vi "CRYUnflatten Scope-FFT.vi"(11 "Flat Scope-FFT setup":string) -> (0 "Error?":bool=TRUE, 2 "Scope-FFT settings":T1={"window"=0, "n avgs"=0, "lin/exp avg"=0, "pwr/cplx avg"=0, "time (ms)"=0.0, "fft lines"=2048, "scope/fft mode"=0, "channel"=0, "trig. channel"=0, "Applay Correction"=FALSE, "Time Display"="%#_6p", "Freq. Weighting"="%.1f", "Ave/Max/Min"=0, "Trigger Level"=0.0, "Trigger Unit"=0, "Trigger Time Offset"=0.0, "Trigger Slope"=0, "Trigger/Free Run"=FALSE, "continuous"=FALSE, "Spectrum Display"="%#_6p", "Calc FFT"=FALSE, "Y-axis"="None", "Signal Type"=""} {"Trigger Time Offset" format="%.2f"; "Trigger Level" format="%.2f"; "time (ms)" format="%.2f"}, 3 "Header info":T2={"Data type"="Data            ", "Version"=1, "Dimensions"=0})   [LabVIEW 2013]
uses:
  Typedef Control/CRYScope-FFT.ctl
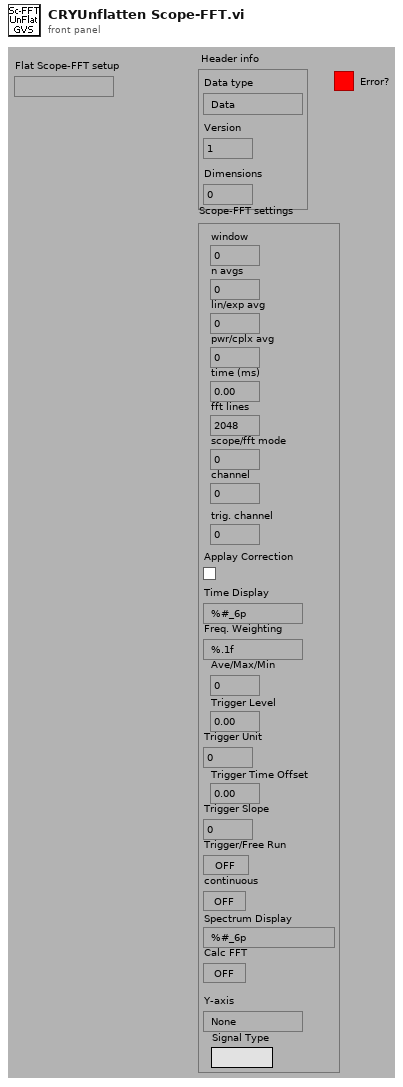
[diagram p1: front panel]
types:
  T1 = typedef "CRYScope-FFT.ctl" = cluster{"window":i32, "n avgs":i32, "lin/exp avg":i32, "pwr/cplx avg":i32, "time (ms)":dbl, "fft lines":i32, "scope/fft mode":i32, "channel":i32, "trig. channel":i32, "Applay Correction":bool, "Time Display":string, "Freq. Weighting":string, "Ave/Max/Min":u16, "Trigger Level":dbl, "Trigger Unit":u16, "Trigger Time Offset":dbl, "Trigger Slope":u16, "Trigger/Free Run":bool, "continuous":bool, "Spectrum Display":string, "Calc FFT":bool, "Y-axis":string, "Signal Type":string}
  T2 = cluster{"Data type":string, "Version":u16, "Dimensions":u8}
  T3 = cluster{"unsigned byte array[0]":u8, "unsigned byte array[1]":u8, "unsigned byte array[2]":u8}
  T4 = cluster{"substring":string, u16, "unsigned byte array[2]":u8}
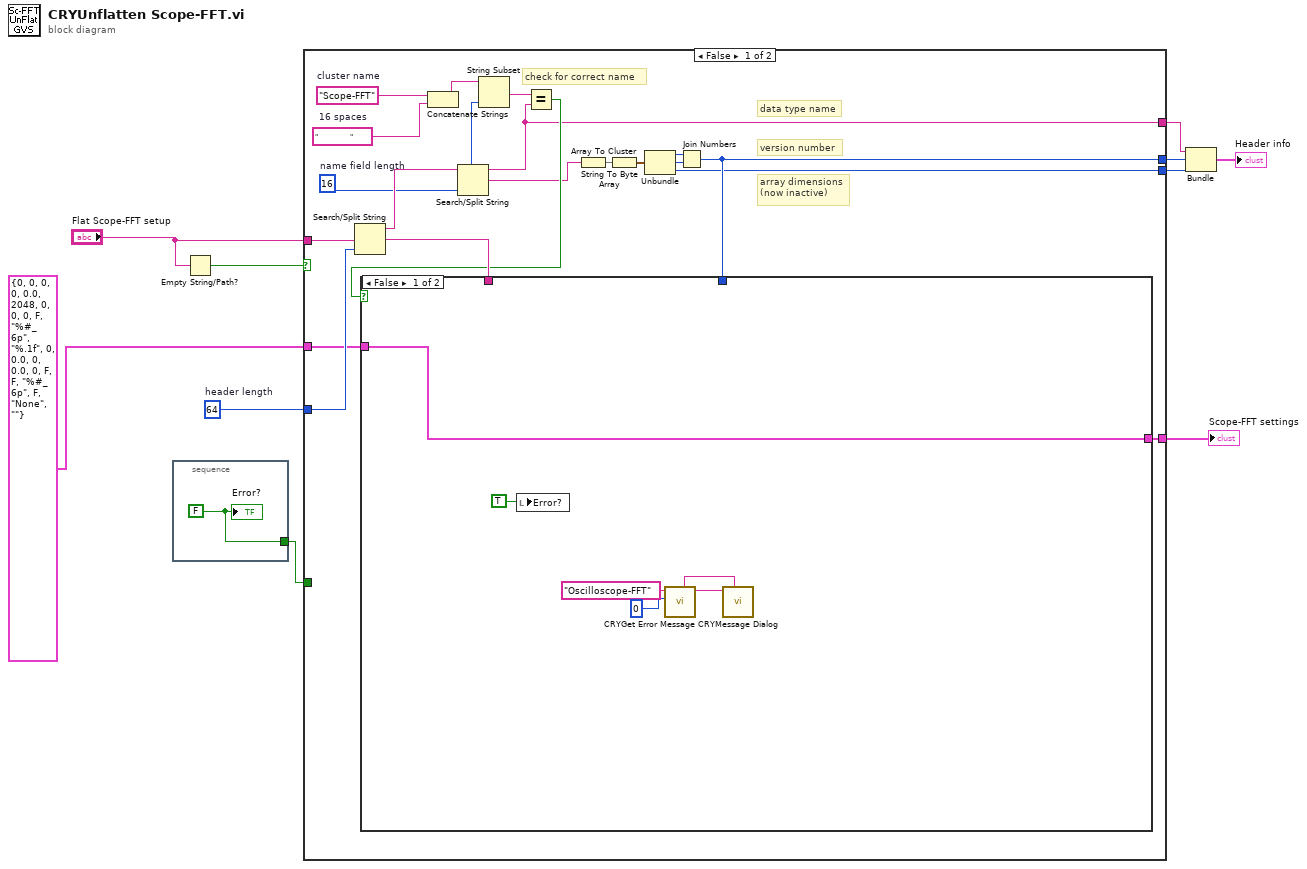
[diagram p0: block diagram]
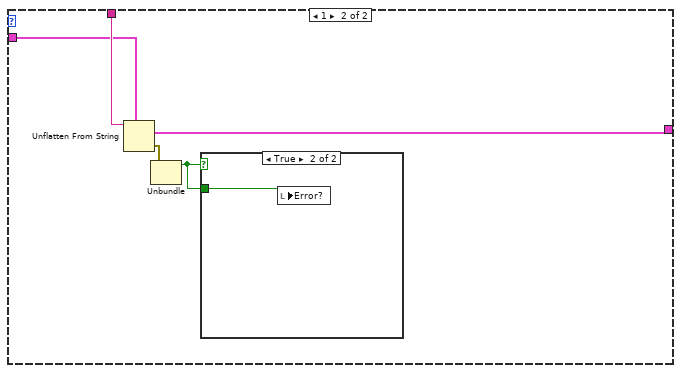
[diagram p3: hidden frame]
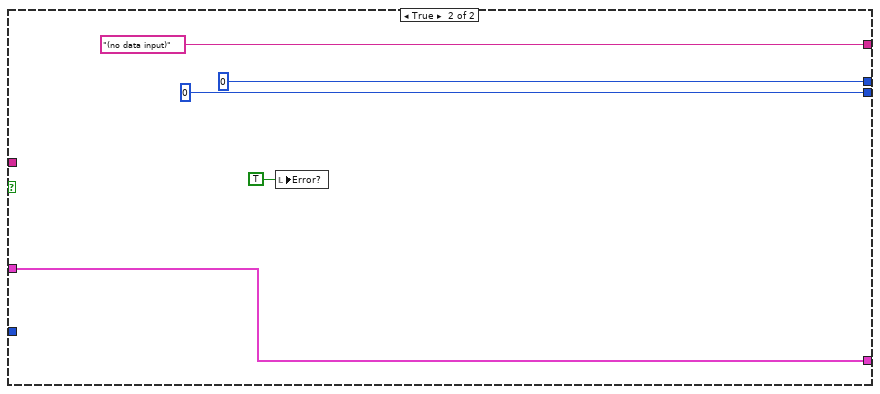
[diagram p5: hidden frame]
diagram:
  w9 = 64  # header length
  n1 = stacked-sequence {
    tunnel: [w11] -> w5
    frame #0 {
      w11 = FALSE
      "Error?" <- w11
    }
  }
  n2 = Empty String/Path?(string/path="Flat Scope-FFT setup") -> (empty?=w10:bool)
  n3 = case shown="False" w10 {
    tunnel: "Flat Scope-FFT setup" -> [w31 _]
    tunnel: w9 -> [w25 _]
    tunnel: [w22 u16 0] -> w7
    tunnel: [w15 u8 0] -> w8
    tunnel: [w16 "(no data input)" ("substring")] -> w6
    tunnel: w5 -> [_ _]
    tunnel: [w14 w49] -> w1
    tunnel: T1 {"window"=0, "n avgs"=0, "lin/exp avg"=0, "pwr/cplx avg"=0, "time (ms)"=0.0, "fft lines"=2048, "scope/fft mode"=0, "channel"=0, "trig. channel"=0, "Applay Correction"=FALSE, "Time Display"="%#_6p", "Freq. Weighting"="%.1f", "Ave/Max/Min"=0, "Trigger Level"=0.0, "Trigger Unit"=0, "Trigger Time Offset"=0.0, "Trigger Slope"=0, "Trigger/Free Run"=FALSE, "continuous"=FALSE, "Spectrum Display"="%#_6p", "Calc FFT"=FALSE, "Y-axis"="None", "Signal Type"=""} ("Scope-FFT settings") -> [w13 w49]
    frame False {
      w12 = "Scope-FFT"  # cluster name
      w20 = "                "  # 16 spaces
      w18 = 16  # name field length
      # "check for correct name"
      # "array dimensions\n(now inactive)"
      # "version number"
      # "data type name"
      n4 = Search/Split String(string=w31, offset (0)=w25) -> (substring before match=w24:string, match + rest of string=w26:string)  [unwired: 2 out]
      n5 = Concatenate Strings(w12, w20) -> (w19:string)
      n6 = Search/Split String(string=w24, offset (0)=w18) -> (substring before match=w16:string, match + rest of string=w21:string)  [unwired: 2 out]
      n7 = String Subset(string=w19, length (rest)=w18) -> (substring=w17:string)  [unwired: 1 out]
      n8 = Equal?(x=w17, y=w16) -> (x = y?=w23:bool)
      n9 = String To Byte Array(string=w21) -> (unsigned byte array=w30:u8[])
      n10 = Array To Cluster(array=w30) -> (cluster=w29:T3)
      n11 = Unbundle(w29) -> ("unsigned byte array[0]"=w28:u8, "unsigned byte array[1]"=w27:u8, "unsigned byte array[2]"=w15:u8)
      n12 = Join Numbers(hi=w28, lo=w27) -> ((hi.lo)=w22:u16)
      n13 = case shown="False" w23 {
        tunnel: w26 -> [_ w41]
        tunnel: w22 -> [_ w40]
        tunnel: [w36 w39] -> w14
        tunnel: w13 -> [w36 w38]
        frame False {
          n14 = local write "Error?"(TRUE) -> ()
          n15 = call "CRYGet Error Message.vi"("Error No"=0, "Kind"="Oscilloscope-FFT") -> ("Message"=w33:string, "Window Title"=w32:string)  [unwired: 4 in, 4 out]
          n16 = call "CRYMessage Dialog.vi"("Window Title"=w32, "Message Content"=w33) -> ()  [unwired: 8 in, 2 out]
        }
        frame True {
          n17 = case "version" shown="Default" w40 {
            tunnel: w41 -> [_ w47]
            tunnel: [w42 w43] -> w39
            tunnel: w38 -> [w42 w44]
            frame Default {
            }
            frame 1 {
              n18 = Unflatten From String(type=w44, binary string=w47) -> (value=w43:T1, error out=w45:errorcluster)  [unwired: 1 in, 3 out]
              n19 = Unbundle(w45) -> ("status"=w46:bool)  [unwired: 2 out]
              n20 = case shown="True" w46 {
                tunnel: w46 -> [_ w48]
                frame False {
                }
                frame True {
                  n21 = local write "Error?"(w48) -> ()
                }
              }
            }
          }
        }
      }
    }
    frame True {
      n22 = local write "Error?"(TRUE ("Error?")) -> ()
    }
  }
  "Scope-FFT settings" <- w1
  n23 = Bundle("substring"=w6, w7, "unsigned byte array[2]"=w8) -> (→"Header info":T4)  [unwired: 1 out]
